vi "Get Connector Pane Info.vi"(8 "Error In":errorcluster, 11 "VI Ref":refnum<vi>) -> (0 "Error Out":errorcluster, 3 "FP Data":T1)   [LabVIEW 2020, in "LMH-Toolbox.lvlib" / "LMH-Front-Panel-Clean-Up.lvlib"]
uses:
  LMH-Front-Panel-Clean-Up.lvlib
  Type Defs/FP Data.ctl
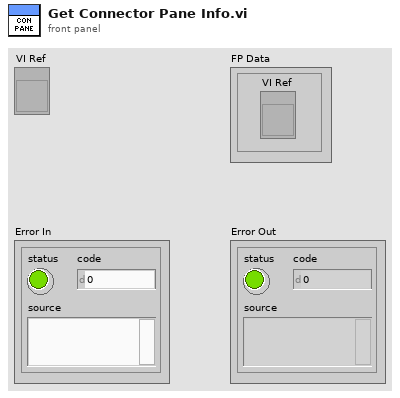
[diagram p1: front panel]
types:
  T1 = typedef "LMH-Toolbox.lvlib/LMH-Front-Panel-Clean-Up.lvlib/FP Data.ctl" = cluster{"VI Ref":refnum<vi>, "FP Objects":refnum<vi>[][], "FP Object Names":string[][], "Max Widths":u32[], "Max Heights":u32[]}
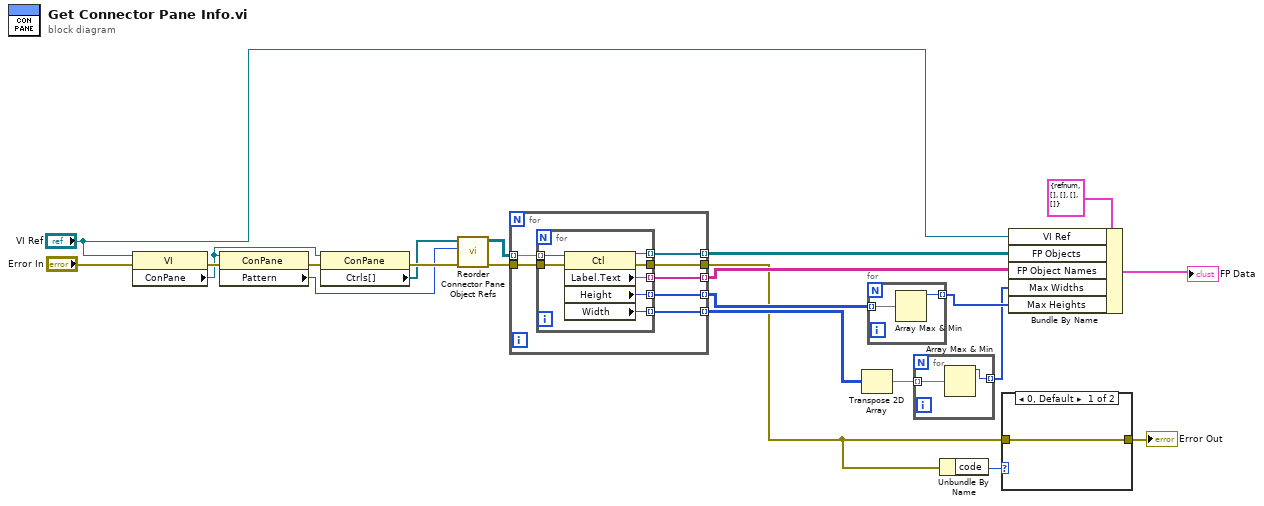
[diagram p0: block diagram]
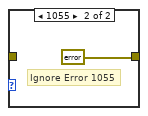
[diagram p2: hidden frame]
diagram:
  n1 = property class="VI"(reference="VI Ref", error in="Error In") -> (error out=w17:errorcluster, "ConPane"=w15:refnum<vi>)  [unwired: 1 out]
  n2 = property class="ConPane"(reference=w15, error in=w17) -> (error out=w18:errorcluster, "Pattern"=w16:u32)  [unwired: 1 out]
  n3 = property class="ConPane"(reference=w15, error in=w18) -> (error out=w19:errorcluster, "Ctrls[]"=w4:refnum<vi>[])  [unwired: 1 out]
  n4 = call "Reorder Connector Pane Object Refs.vi"("Error In"=w19, "Connector Pane Patter"=w16, "Connector Pane Object Refs"=w4) -> ("Error Out"=w1:errorcluster, "Connector Pane Object Refs"=w2:refnum<vi>[][])  [unwired: 7 in]
  n5 = for {
    tunnel: [w27] -> w11 mode=indexing
    tunnel: [w26] -> w20 mode=indexing
    tunnel: [w25] -> w21 mode=indexing
    tunnel: w1 -> [w29]
    tunnel: [w28] -> w5
    tunnel: w2 -> [w24] mode=indexing
    tunnel: [w23] -> w3 mode=indexing
    n6 = for {
      tunnel: [w34] -> w27 mode=indexing
      tunnel: [w33] -> w26 mode=indexing
      tunnel: [w32] -> w25 mode=indexing
      tunnel: w29 -> [w36]
      tunnel: [w35] -> w28
      tunnel: w24 -> [w31] mode=indexing
      tunnel: [w30] -> w23 mode=indexing
      n7 = property class="Ctl"(reference=w31, error in=w36) -> (reference out=w30:refnum<vi>, error out=w35:errorcluster, "Label.Text"=w34:string, "Height"=w33:u32, "Width"=w32:u32)
    }
  }
  n8 = Transpose 2D Array(2D array=w21) -> (transposed array=w22:u32[][])
  n9 = for {
    tunnel: [w38] -> w13 mode=indexing
    tunnel: w20 -> [w37] mode=indexing
    n10 = Array Max & Min(array=w37) -> (max value=w38:u32)  [unwired: 3 out]
  }
  n11 = for {
    tunnel: [w40] -> w12 mode=indexing
    tunnel: w22 -> [w39] mode=indexing
    n12 = Array Max & Min(array=w39) -> (max value=w40:u32)  [unwired: 3 out]
  }
  n13 = Unbundle By Name(w5) -> ("code"=w7:i32)
  n14 = case shown="0, Default" w7 {
    tunnel: [w41 errorcluster {"status"=FALSE, "code"=0, "source"=""} ("error out")] -> w6
    tunnel: w5 -> [w41 _]
    frame 0, Default {
    }
    frame 1055 {
      # "Ignore Error 1055"
    }
  }
  "Error Out" <- w6
  n15 = Bundle By Name(cluster=T1 {"VI Ref"=refnum, "FP Objects"=[], "FP Object Names"=[], "Max Widths"=[], "Max Heights"=[]} ("FP Data"), "VI Ref"="VI Ref", "FP Objects"=w3, "FP Object Names"=w11, "Max Widths"=w12, "Max Heights"=w13) -> (→"FP Data":T1)
